vi "Rotation Matrix.vi"(11 "Rotation":T2) -> (3 "Rxyz":T1 format="%#.6f")   [LabVIEW 2020]
uses:
  Vec3.ctl
  <vilib>/Analysis/Matrix/Datatypes/RealMatrix.ctl
  <vilib>/Analysis/Matrix/Numeric/Multiply/Multiply - RM,R.vi
  <vilib>/Analysis/Matrix/Numeric/Add/Add - RM,RM.vi
  <vilib>/Analysis/Matrix/Numeric/Multiply/Multiply - RM,RM.vi
  <vilib>/Analysis/Matrix/NI_Matrix.lvlib
panel:
  out "Rz":T1 format="%#.6f"
  out "Ry":T1 format="%#.6f"
  out "Rx":T1 format="%#.6f"
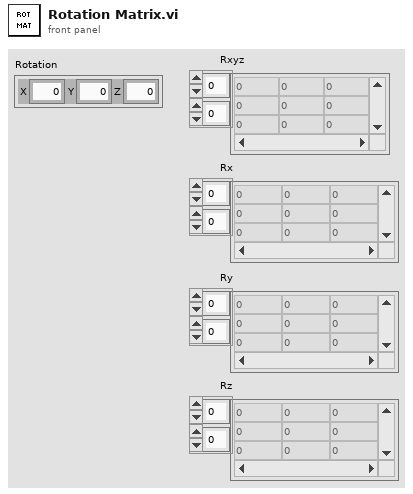
[diagram p1: front panel]
types:
  T1 = typedef "NI_Matrix.lvlib/RealMatrix.ctl" = dbl[][]
  T2 = typedef "Vec3.ctl" = cluster{"X":dbl, "Y":dbl, "Z":dbl}
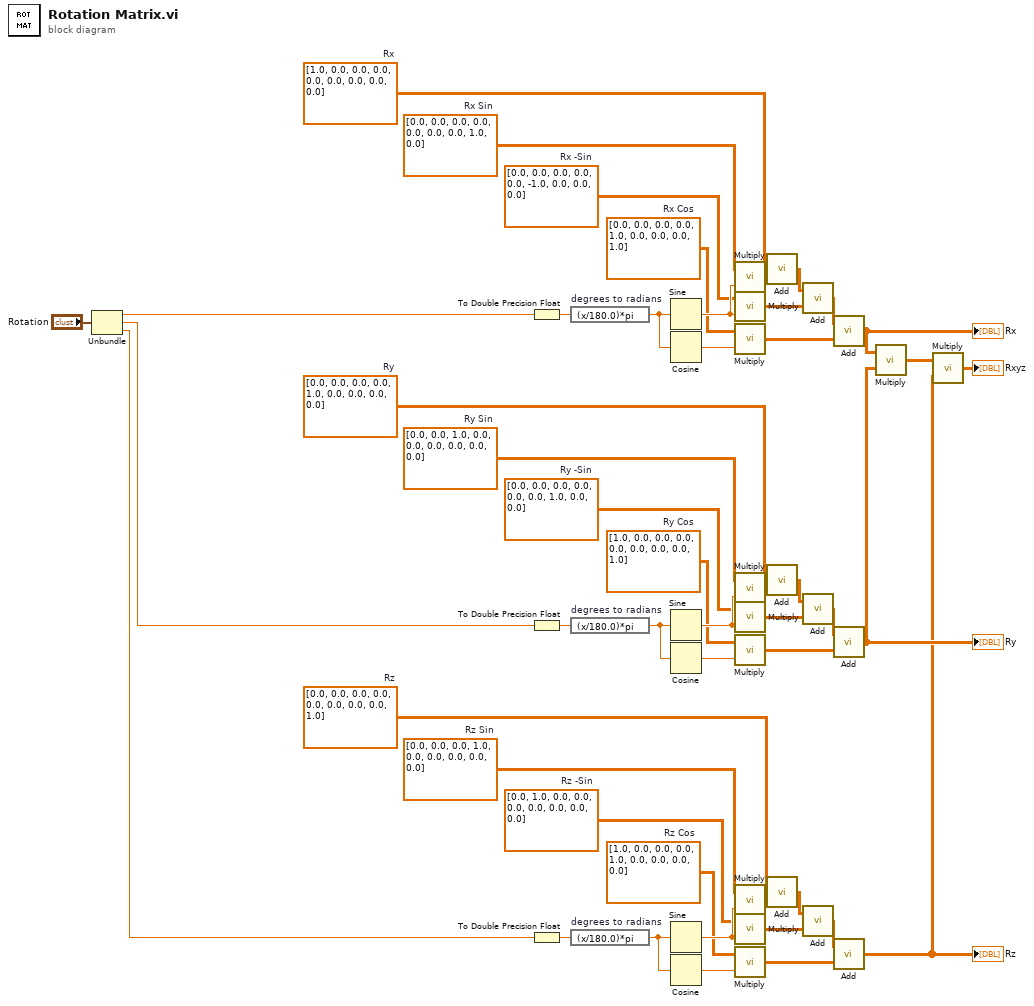
[diagram p0: block diagram]
diagram:
  w7 = T1 [[0.0, 0.0, 0.0], [0.0, 0.0, 0.0], [0.0, 0.0, 1.0]]  # Rz
  w10 = T1 [[1.0, 0.0, 0.0], [0.0, 1.0, 0.0], [0.0, 0.0, 0.0]]  # Rz Cos
  w8 = T1 [[0.0, 0.0, 0.0], [1.0, 0.0, 0.0], [0.0, 0.0, 0.0]]  # Rz Sin
  w9 = T1 [[0.0, 1.0, 0.0], [0.0, 0.0, 0.0], [0.0, 0.0, 0.0]]  # Rz -Sin
  w22 = T1 [[0.0, 0.0, 0.0], [0.0, 1.0, 0.0], [0.0, 0.0, 0.0]]  # Ry
  w19 = T1 [[1.0, 0.0, 0.0], [0.0, 0.0, 0.0], [0.0, 0.0, 1.0]]  # Ry Cos
  w21 = T1 [[0.0, 0.0, 1.0], [0.0, 0.0, 0.0], [0.0, 0.0, 0.0]]  # Ry Sin
  w20 = T1 [[0.0, 0.0, 0.0], [0.0, 0.0, 0.0], [1.0, 0.0, 0.0]]  # Ry -Sin
  w34 = T1 [[1.0, 0.0, 0.0], [0.0, 0.0, 0.0], [0.0, 0.0, 0.0]]  # Rx
  w36 = T1 [[0.0, 0.0, 0.0], [0.0, 1.0, 0.0], [0.0, 0.0, 1.0]]  # Rx Cos
  w40 = T1 [[0.0, 0.0, 0.0], [0.0, 0.0, 0.0], [0.0, 1.0, 0.0]]  # Rx Sin
  w38 = T1 [[0.0, 0.0, 0.0], [0.0, 0.0, -1.0], [0.0, 0.0, 0.0]]  # Rx -Sin
  n1 = Unbundle("Rotation") -> ("X"=w47:dbl, "Y"=w43:dbl, "Z"=w42:dbl)
  n2 = To Double Precision Float(number=w47) -> (double precision float=w46:dbl)
  n3 = To Double Precision Float(number=w43) -> (double precision float=w45:dbl)
  n4 = To Double Precision Float(number=w42) -> (double precision float=w44:dbl)
  n5 = expression code="(x/180.0)*pi" "degrees to radians"(w46) -> (w48:dbl)
  n6 = expression code="(x/180.0)*pi" "degrees to radians"(w45) -> (w6:dbl)
  n7 = expression code="(x/180.0)*pi" "degrees to radians"(w44) -> (w11:dbl)
  n8 = Sine(x=w48) -> (sin(x)=w39:dbl)
  n9 = Cosine(x=w48) -> (cos(x)=w37:dbl)
  n10 = Sine(x=w6) -> (sin(x)=w23:dbl)
  n11 = Cosine(x=w6) -> (cos(x)=w24:dbl)
  n12 = Sine(x=w11) -> (sin(x)=w18:dbl)
  n13 = Cosine(x=w11) -> (cos(x)=w17:dbl)
  n14 = call-poly <vilib>:"Multiply.vi"("Real Scalar c"=w39, "Real Matrix A"=w40) -> ("A * c"=w35:T1)
  n15 = call-poly <vilib>:"Multiply.vi"("Real Scalar c"=w39, "Real Matrix A"=w38) -> ("A * c"=w33:T1)
  n16 = call-poly <vilib>:"Multiply.vi"("Real Scalar c"=w37, "Real Matrix A"=w36) -> ("A * c"=w31:T1)
  n17 = call-poly <vilib>:"Multiply.vi"("Real Scalar c"=w23, "Real Matrix A"=w21) -> ("A * c"=w25:T1)
  n18 = call-poly <vilib>:"Multiply.vi"("Real Scalar c"=w23, "Real Matrix A"=w20) -> ("A * c"=w26:T1)
  n19 = call-poly <vilib>:"Multiply.vi"("Real Scalar c"=w24, "Real Matrix A"=w19) -> ("A * c"=w28:T1)
  n20 = call-poly <vilib>:"Multiply.vi"("Real Scalar c"=w18, "Real Matrix A"=w8) -> ("A * c"=w16:T1)
  n21 = call-poly <vilib>:"Multiply.vi"("Real Scalar c"=w18, "Real Matrix A"=w9) -> ("A * c"=w15:T1)
  n22 = call-poly <vilib>:"Multiply.vi"("Real Scalar c"=w17, "Real Matrix A"=w10) -> ("A * c"=w13:T1)
  n23 = call-poly <vilib>:"Add.vi"("Real Matrix B"=w35, "Real Matrix A"=w34) -> ("A + B"=w32:T1)
  n24 = call-poly <vilib>:"Add.vi"("Real Matrix B"=w25, "Real Matrix A"=w22) -> ("A + B"=w27:T1)
  n25 = call-poly <vilib>:"Add.vi"("Real Matrix B"=w16, "Real Matrix A"=w7) -> ("A + B"=w14:T1)
  n26 = call-poly <vilib>:"Add.vi"("Real Matrix B"=w33, "Real Matrix A"=w32) -> ("A + B"=w30:T1)
  n27 = call-poly <vilib>:"Add.vi"("Real Matrix B"=w26, "Real Matrix A"=w27) -> ("A + B"=w29:T1)
  n28 = call-poly <vilib>:"Add.vi"("Real Matrix B"=w15, "Real Matrix A"=w14) -> ("A + B"=w12:T1)
  n29 = call-poly <vilib>:"Add.vi"("Real Matrix B"=w31, "Real Matrix A"=w30) -> ("A + B"=w5:T1)
  "Rx" <- w5
  n30 = call-poly <vilib>:"Add.vi"("Real Matrix B"=w28, "Real Matrix A"=w29) -> ("A + B"=w4:T1)
  "Ry" <- w4
  n31 = call-poly <vilib>:"Add.vi"("Real Matrix B"=w13, "Real Matrix A"=w12) -> ("A + B"=w2:T1)
  "Rz" <- w2
  n32 = call-poly <vilib>:"Multiply.vi"("Real Matrix B"=w4, "Real Matrix A"=w5) -> ("A * B"=w3:T1)
  n33 = call-poly <vilib>:"Multiply.vi"("Real Matrix B"=w2, "Real Matrix A"=w3) -> ("A * B"=→"Rxyz":T1)
